vi "ALTER ITEM DESCRIPTION.vi"(10 "REFERENCES":T2, 11 "DATA IN":T1[](array[typedef])) -> (3 "DATA OUT":T1[](array[typedef]))   [LabVIEW 2019]
uses:
  Controls/Table Data Types/Inventory Data Type.ctl
  Controls/References Cluster.ctl
  <vilib>/userDefined/High Color/IMAQdx.ctl
  Controls/Custom Calendar/Custom Calendar.xctl
  <vilib>/regexp/Match Regular Expression.xnode
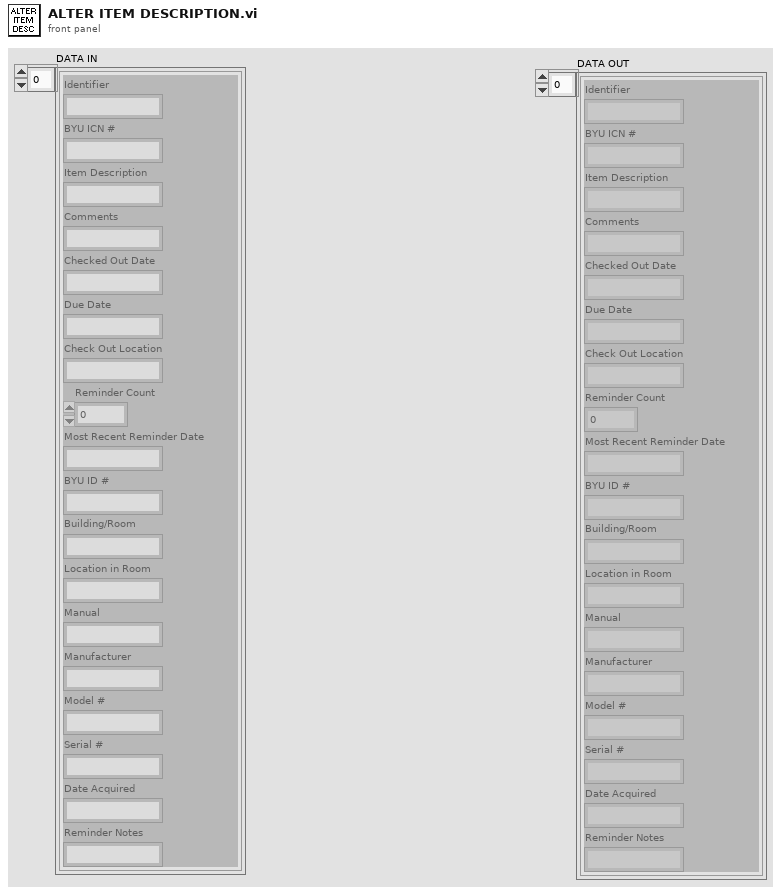
[diagram p1: front panel]
types:
  T1 = typedef "Inventory Data Type.ctl" = cluster{"Identifier":string, "BYU ICN #":string, "Item Description":string, "Comments":string, "Checked Out Date":string, "Due Date":string, "Check Out Location":string, "Reminder Count":i32, "Most Recent Reminder Date":string, "BYU ID #":string, "Building/Room":string, "Location in Room":string, "Manual":string, "Manufacturer":string, "Model #":string, "Serial #":string, "Date Acquired":string, "Reminder Notes":string}
  T2 = typedef "References Cluster.ctl" = cluster{"MAIN PAGES":refnum<vi>, "ADD/EDIT ITEM REFERENCES":cluster{"Identifier":refnum<vi>, "BYU ICN #":refnum<vi>, "Item Description":refnum<vi>, "Comments":refnum<vi>, "Checked Out Date":refnum<vi>, "Due Date":refnum<vi>, "Check Out Location":refnum<vi>, "Reminder Count":refnum<vi>, "Most Recent Reminder Date":refnum<vi>, "BYU ID #":refnum<vi>, "Building/Room":refnum<vi>, "Location in Room":refnum<vi>, "Manual":refnum<vi>, "Manufacturer":refnum<vi>, "Model #":refnum<vi>, "Serial #":refnum<vi>, "Date Acquired":refnum<vi>, "ADD/EDIT ITEM LABEL":refnum<vi>, "ARCHIVE ITEM":refnum<vi>, "Archive Item Inputs":refnum<vi>, "Reminder Notes":refnum<vi>, "DUPLICATE ITEM":refnum<vi>}, "ADD/EDIT USER REFERENCES":cluster{"BYU ID # (##-###-####)":refnum<vi>, "First Name":refnum<vi>, "Last Name":refnum<vi>, "Phone Number (###-###-####)":refnum<vi>, "Email":refnum<vi>, "Department":refnum<vi>, "Graduation Status":refnum<vi>, "Anticipated Graduation Year":refnum<vi>, "Credit Score":refnum<vi>, "Date Added":refnum<vi>, "Graduation Clearance Date":refnum<vi>, "Picture File Name":refnum<vi>, "ADD/EDIT USER LABEL":refnum<vi>, "Department Map":refnum<vi>, "Status Map":refnum<vi>, "Anticipated Graduation Year Map":refnum<vi>, "User Agreement":refnum<vi>, "User Comments":refnum<vi>, "Camera":refnum<vi>}, "RETURN ITEM REFERENCES":cluster{"Item or Person:":refnum<vi>, "Search Return Results":refnum<vi>, "What are you searching for?":refnum<vi>}, "SEARCH DATABASE REFERENCES":cluster{"What to Search For:":refnum<vi>, "Where to Search":refnum<vi>, "Column to Search In":refnum<vi>, "Column to Sort By":refnum<vi>, "Search Database Results":refnum<vi>, "Inventory Column Selector":refnum<vi>, "User Column Selector":refnum<vi>, "Inventory Archive Column Selector":refnum<vi>, "User Archive Column Selector":refnum<vi>, "Sales Tracking Column Selector":refnum<vi>, "Checked In Archive Column Selector":refnum<vi>, "Restore User":refnum<vi>, "Date Range":refnum<vi>, "Dates Less Than":refnum<vi>, "Dates Greater Than":refnum<vi>, "Search Print Receipt":refnum<vi>, "Edit Sale Description":refnum<vi>}, "USER ITEMS REFERENCES":cluster{"USER'S INFORMATION":refnum<vi>, "User's Checked Out Items":refnum<vi>, "User Info Comments":refnum<vi>, "SEE USER INFO COMMENTS":refnum<vi>}, "EDIT ITEMS REFERENCES":cluster{"New Check Out Location":refnum<vi>, "Items to Edit":refnum<vi>, "Edit Items Due Date":refnum<vi>, "New Reminder Notes":refnum<vi>, "New Item Description":refnum<vi>}, "CHECK OUT ITEMS REFERENCES":cluster{"Enter Item:":refnum<vi>, "Check Out Items Due Date":refnum<vi>, "Check Out Location":refnum<vi>, "Items to be Checked Out":refnum<vi>, "Possible Items":refnum<vi>, "Altered Item Description":refnum<vi>}, "TRANSFER ITEMS REFERENCES":cluster{"Search Parameter":refnum<vi>, "What to Match":refnum<vi>, "Matching Individuals":refnum<vi>, "Items to be Transferred":refnum<vi>}, "SETTINGS REFERENCES":cluster{"PSC Database Settings":refnum<vi>, "PSC Sales Item Spreadsheet":refnum<vi>}, "PSC SALES REFERENCES":cluster{"BYU ID CARD #":refnum<vi>, "Sale Description":refnum<vi>, "Scan or Enter Item Name":refnum<vi>, "Items to be Sold":refnum<vi>, "Grand Total":refnum<vi>, "Item List":refnum<vi>}}
  T3 = cluster{"Enter Item:":refnum<vi>, "Check Out Items Due Date":refnum<vi>, "Check Out Location":refnum<vi>, "Items to be Checked Out":refnum<vi>, "Possible Items":refnum<vi>, "Altered Item Description":refnum<vi>}
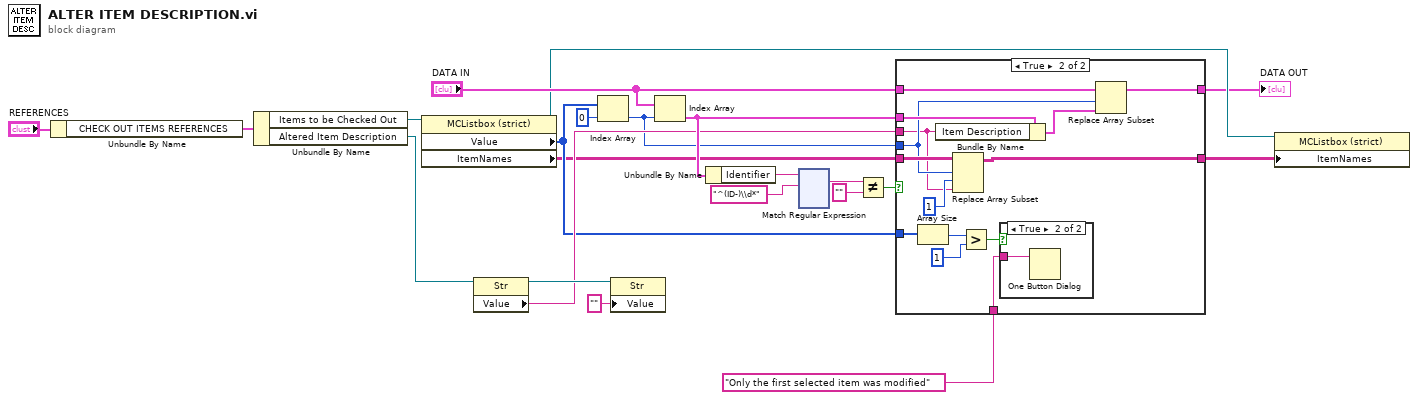
[diagram p0: block diagram]
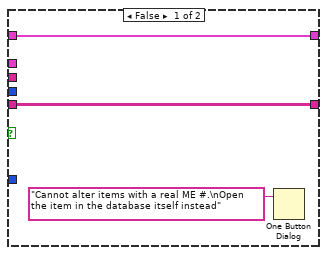
[diagram p2: hidden frame]
diagram:
  n1 = Unbundle By Name("REFERENCES") -> ("CHECK OUT ITEMS REFERENCES"=w21:T3)
  n2 = Unbundle By Name(w21) -> ("Items to be Checked Out"=w20:refnum<vi>, "Altered Item Description"=w19:refnum<vi>)
  n3 = property class="MCListbox (strict)"(reference=w20) -> (reference out=w4:refnum<vi>, "Value"=w7:i32[], "ItemNames"=w5:string[][])  [unwired: 1 in, 1 out]
  n4 = property class="Str"(reference=w19) -> (reference out=w17:refnum<vi>, "Value"=w9:string)  [unwired: 1 in, 1 out]
  n5 = Index Array(array=w7, index=0) -> (element=w3:i32)
  n6 = property class="Str"(reference=w17, "Value"="") -> ()  [unwired: 1 in, 2 out]
  n7 = Index Array(array="DATA IN", index=w3) -> (element=w10:T1)
  n8 = Unbundle By Name(w10) -> ("Identifier"=w12:string)
  n9 = xnode "Match Regular Expression"("input string"=w12, "regular expression"="^(ID-)\\d*") -> ("whole match"=w14:string)  [unwired: 4 in, 4 out]
  n10 = Not Equal?(x=w14, y="") -> (x != y?=w11:bool)
  n11 = case shown="True" w11 {
    tunnel: w10 -> [_ w39]
    tunnel: w9 -> [_ w28]
    tunnel: "DATA IN" -> [w24 w38]
    tunnel: w7 -> [_ w35]
    tunnel: "Only the first selected item was modified" ("message") -> [_ w33]
    tunnel: w5 -> [w23 w31]
    tunnel: w3 -> [_ w30]
    tunnel: [w23 w27] -> w2
    tunnel: [w24 w26] -> w1
    frame False {
      n12 = One Button Dialog(message="Cannot alter items with a real ME #.\nOpen the item in the database itself instead") -> ()  [unwired: 1 in, 1 out]
    }
    frame True {
      n13 = Array Size(array=w35) -> (size(s)=w37:i32)
      n14 = Bundle By Name(cluster=w39, "Item Description"=w28) -> (w32:T1)
      n15 = Replace Array Subset(array=w31, new element=w28, index (row)=w30, index (col)=1 ("disabled index (col)")) -> (w27:string[][])
      n16 = Greater?(x=w37, y=1) -> (0:w34:bool)
      n17 = case shown="True" w34 {
        tunnel: w33 -> [_ w40]
        frame False {
        }
        frame True {
          n18 = One Button Dialog(message=w40) -> ()  [unwired: 1 in, 1 out]
        }
      }
      n19 = Replace Array Subset(array=w38, new element=w32, index=w30) -> (w26:T1[])
    }
  }
  "DATA OUT" <- w1
  n20 = property class="MCListbox (strict)"(reference=w4, "ItemNames"=w2) -> ()  [unwired: 1 in, 2 out]
